vi "StopStacking.vi"(11 "Array":bool[](array[boolean])) -> ()   [LabVIEW 2014]
uses:
  StopStacking.ctl
  AutomationGlobals.vi
  Gantry/GantryGlobals.vi
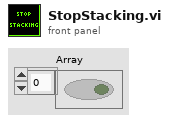
[diagram p1: front panel]
types:
  T1 = typedef "StopStacking.ctl" = enum16{"WaitingForInput", "DisableAutoStack", "LowerLift", "OpenArms", "CloseCanGrabbers", "RaiseLift", "CloseArms"}
  T2 = typedef "WPI_SwitchDevRef.ctl" = cluster{"DevStatus":errorcluster, "DIO Channel":T3, "Controller":T4, "CntIndex":T5, "Normally Closed":bool}
  T3 = typedef "FPGA_DIOChannel.ctl" = enum8{"DIO 0", "DIO 1", "DIO 2", "DIO 3", "DIO 4", "DIO 5", "DIO 6", "DIO 7", "DIO 8", "DIO 9", "DIO MXP 0", "DIO MXP 1", "DIO MXP 2", "DIO MXP 3", "DIO MXP 4", "DIO MXP 5", "DIO MXP 6", "DIO MXP 7", "DIO MXP 8", "DIO MXP 9", "DIO MXP 10", "DIO MXP 11", "DIO MXP 12", "DIO MXP 13", "DIO MXP 14", "DIO MXP 15", "Invalid"}
  T4 = typedef "FPGA_TypedefDigitalModule.ctl" = enum16{"Controller 1"}
  T5 = typedef "FPGA_CounterCtrSystemIndex.ctl" = enum8{"Ctr 0", "Ctr 1", "Ctr 2", "Ctr 3", "Ctr 4", "Ctr 5", "Ctr 6", "Ctr 7", "Invalid"}
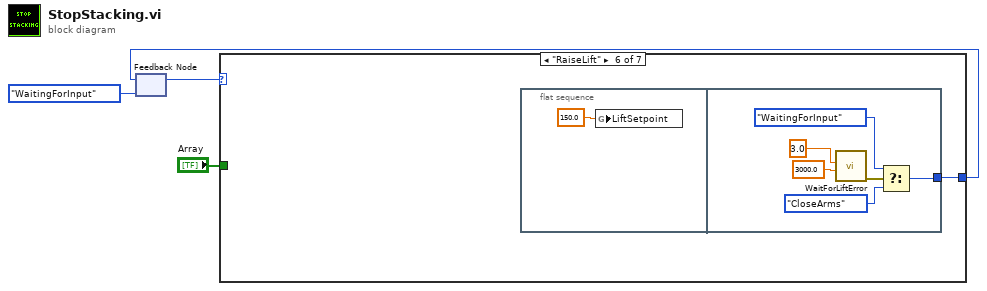
[diagram p0: block diagram]
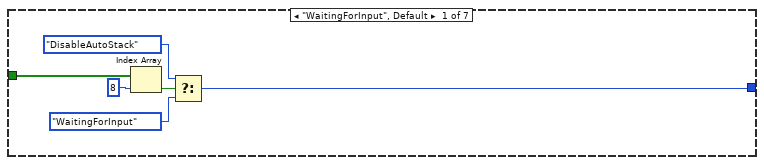
[diagram p2: hidden frame]
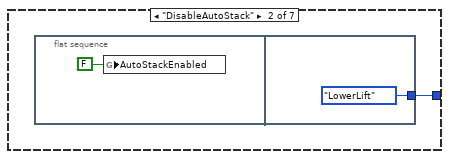
[diagram p3: hidden frame]
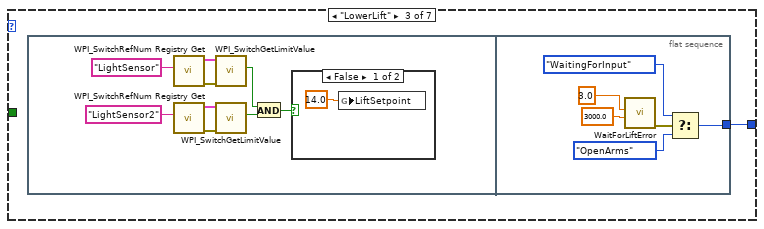
[diagram p4: hidden frame]
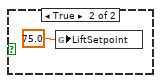
[diagram p5: hidden frame]
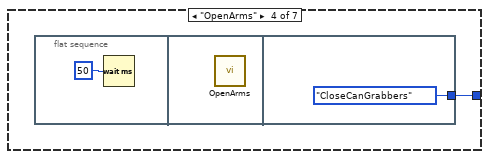
[diagram p6: hidden frame]
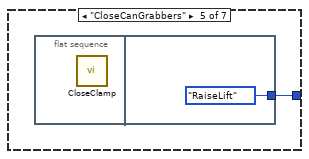
[diagram p7: hidden frame]
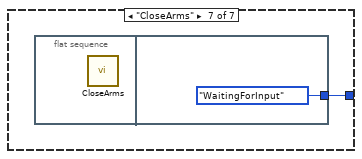
[diagram p8: hidden frame]
diagram:
  n1 = feedback #1(StopStacking."WaitingForInput" ("Enum")) -> (w3:T1)
  n2 = case shown="\"RaiseLift\"" w3 {
    tunnel: "Array" -> [w9 _ _ _ _ _ _]
    tunnel: [w5 w11 w14 w32 w35 w37 w45] -> w1
    frame "WaitingForInput", Default {
      n3 = Index Array(array=w9, index=8) -> (element=w8:bool)
      n4 = Select(t=StopStacking."DisableAutoStack" ("Enum"), s=w8, f=StopStacking."WaitingForInput" ("Enum")) -> (s? t:f=w5:T1)
    }
    frame "DisableAutoStack" {
      n5 = flat-sequence {
        tunnel: [StopStacking."LowerLift" ("Enum")] -> w11
        frame #0 {
          n6 = global write "AutomationGlobals.vi" "AutoStackEnabled"(FALSE ("AutoStackEnabled")) -> ()
        }
        frame #1 {
        }
      }
    }
    frame "LowerLift" {
      n7 = flat-sequence {
        tunnel: [w28] -> w14
        frame #0 {
          n8 = call <vilib>:"WPI_SwitchRefNum Registry Get.vi"("refnum name"="LightSensor") -> ("error out"=w20:errorcluster, "SwitchDevRef"=w21:T2)  [unwired: 9 in]
          n9 = call <vilib>:"WPI_SwitchRefNum Registry Get.vi"("refnum name"="LightSensor2") -> ("error out"=w19:errorcluster, "SwitchDevRef"=w18:T2)  [unwired: 9 in]
          n10 = call <vilib>:"WPI_SwitchGetLimitValue.vi"("error in (no error)"=w20, "SwitchDevRef"=w21) -> ("Switch Pressed"=w22:bool)  [unwired: 7 in, 2 out]
          n11 = call <vilib>:"WPI_SwitchGetLimitValue.vi"("error in (no error)"=w19, "SwitchDevRef"=w18) -> ("Switch Pressed"=w23:bool)  [unwired: 7 in, 2 out]
          n12 = And(x=w22, y=w23) -> (x .and. y?=w15:bool)
          n13 = case shown="False" w15 {
            frame False {
              n14 = global write "GantryGlobals.vi" "LiftSetpoint"(14.0 ("LiftSetpoint")) -> ()
            }
            frame True {
              n15 = global write "GantryGlobals.vi" "LiftSetpoint"(75.0 ("LiftSetpoint")) -> ()
            }
          }
        }
        frame #1 {
          n16 = call "WaitForLiftError.vi"("Timeout (ms)"=3000.0, "AllowedError"=3.0) -> ("error out"=w31:errorcluster)  [unwired: 9 in]
          n17 = Select(t=StopStacking."WaitingForInput" ("Enum"), s=w31, f=StopStacking."OpenArms" ("Enum")) -> (s? t:f=w28:T1)
        }
      }
    }
    frame "OpenArms" {
      n18 = flat-sequence {
        tunnel: [StopStacking."CloseCanGrabbers" ("Enum")] -> w32
        frame #0 {
          n19 = Wait (ms)(milliseconds to wait=u32 50) -> ()  [unwired: 1 out]
        }
        frame #1 {
          n20 = call "OpenArms.vi"() -> ()  [unwired: 12 in]
        }
        frame #2 {
        }
      }
    }
    frame "CloseCanGrabbers" {
      n21 = flat-sequence {
        tunnel: [StopStacking."RaiseLift" ("Enum")] -> w35
        frame #0 {
          n22 = call "CloseClamp.vi"() -> ()  [unwired: 12 in]
        }
        frame #1 {
        }
      }
    }
    frame "RaiseLift" {
      n23 = flat-sequence {
        tunnel: [w39] -> w37
        frame #0 {
          n24 = global write "GantryGlobals.vi" "LiftSetpoint"(150.0 ("LiftSetpoint")) -> ()
        }
        frame #1 {
          n25 = call "WaitForLiftError.vi"("Timeout (ms)"=3000.0, "AllowedError"=3.0) -> ("error out"=w44:errorcluster)  [unwired: 9 in]
          n26 = Select(t=StopStacking."WaitingForInput" ("Enum"), s=w44, f=StopStacking."CloseArms" ("Enum")) -> (s? t:f=w39:T1)
        }
      }
    }
    frame "CloseArms" {
      n27 = flat-sequence {
        tunnel: [StopStacking."WaitingForInput" ("Enum")] -> w45
        frame #0 {
          n28 = call "CloseArms.vi"() -> ()  [unwired: 12 in]
        }
        frame #1 {
        }
      }
    }
  }
  n29 = feedback-in #1(w1) -> ()
